vi "Log Status.vi"(7 "Context ID":u32, 8 "error in":errorcluster, 9 "Action":T1, 10 "Socket Counter":u32, 11 "Context Counter":u32) -> (0 "error out":errorcluster)   [LabVIEW 2019, in "RemoteControl.ZMQ.lvlib" / "ZMQ.ContextManager.lvlib"]
uses:
  ZMQ.ContextManager.lvlib
  Typedefs/Action--enum.ctl
  <vilib>/Utility/sysdir.llb/System Directory Type.ctl
  <vilib>/Utility/file.llb/Write Delimited Spreadsheet (string).vi
  <vilib>/Utility/config.llb/Read Key (Boolean).vi
  <vilib>/Utility/config.llb/Write Key (Boolean).vi
  <vilib>/Utility/config.llb/NI_LVConfig.lvlib
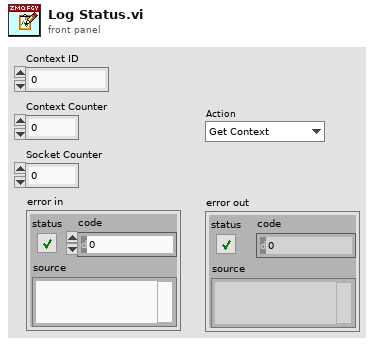
[diagram p1: front panel]
types:
  T1 = typedef "RemoteControl.ZMQ.lvlib/ZMQ.ContextManager.lvlib/Action--enum.ctl" = enum16{"Get Context", "Release Context", "Socket Opened", "Socket Closed", "Force Cleanup"}
  T2 = typedef "System Directory Type.ctl" = i32
  T3 = typedef "NI_LVConfig.lvlib/Config Data RefNum.ctl" = refnum<k1>
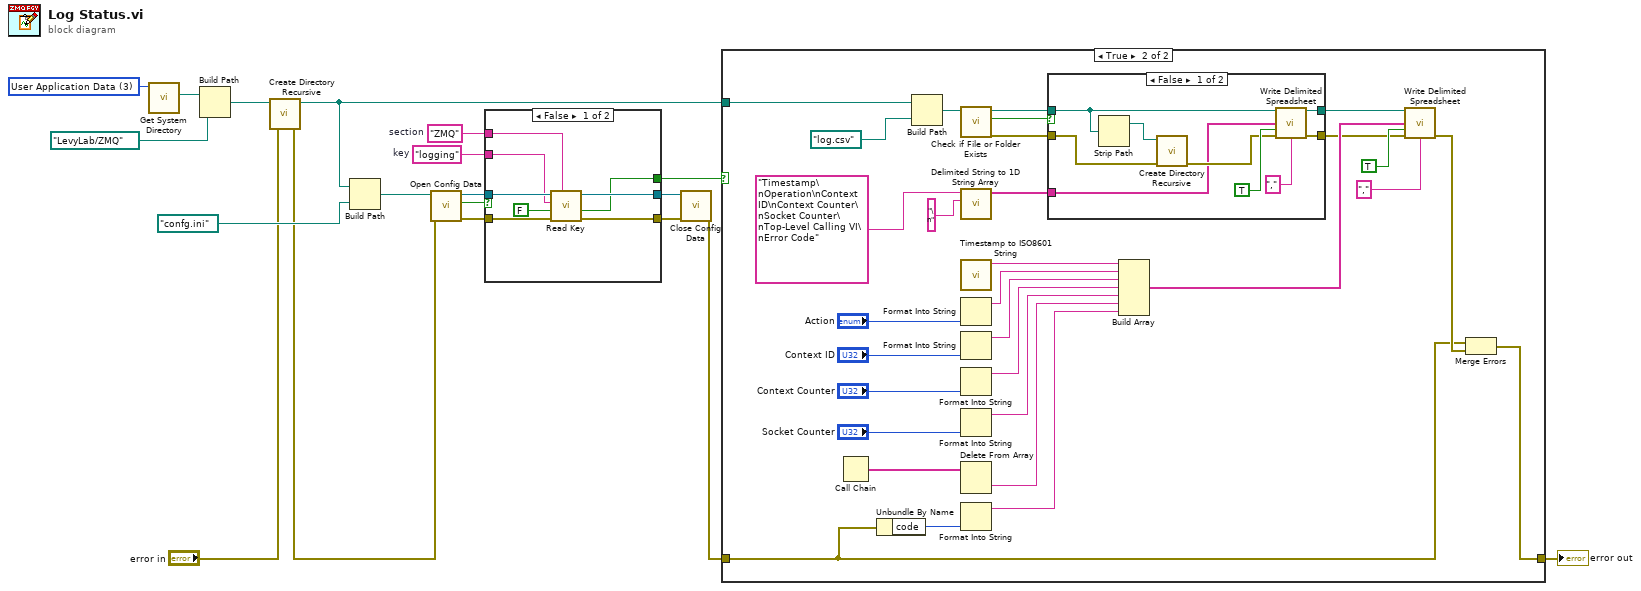
[diagram p0: block diagram]
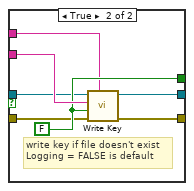
[diagram p2: hidden frame]
diagram:
  w5 = "logging"  # key
  w6 = "ZMQ"  # section
  w19 = T2 3 items=["User Home"=0, "User Desktop"=1, "User Documents"=2, "User Application Data"=3, "User Preferences"=4, "User Temporary"=5, "Public Documents"=6, "Public Application Data"=7, "Public Preferences"=8, "Public Cache"=13, "System Core Libraries"=9, "System Installed Libraries"=10, "Application Files"=11, "Boot Volume Root"=12] ("system directory type")
  n1 = call <vilib>:"Get System Directory.vi"("system directory type"=w19) -> ("system directory"=w18:path)  [unwired: 10 in]
  n2 = Build Path(base path=w18, name or relative path=path "LevyLab/ZMQ") -> (appended path=w4:path)
  n3 = call <vilib>:"Create Directory Recursive.vi"("error in (no error)"="error in", "directory"=w4) -> ("error out"=w1:errorcluster, "directory copy"=w3:path)  [unwired: 3 in, 1 out]
  n4 = Build Path(base path=w3, name or relative path=path "confg.ini") -> (appended path=w15:path)
  n5 = call <vilib>:"Open Config Data.vi"("error in (no error)"=w1, "configuration file path"=w15) -> ("error out"=w13:errorcluster, "file created?"=w7:bool, "refnum"=w14:T3)  [unwired: 7 in]
  n6 = case shown="False" w7 {
    tunnel: w14 -> [w27 w29]
    tunnel: w13 -> [w26 w28]
    tunnel: [w24 w32] -> w11
    tunnel: [w23 w31] -> w10
    tunnel: [w22 w33] -> w8
    tunnel: w6 -> [w21 w30]
    tunnel: w5 -> [w20 w34]
    frame False {
      n7 = call-poly <vilib>:"Read Key.vi"("section"=w21, "error in (no error)"=w26, "default value"=FALSE, "key"=w20, "refnum"=w27) -> ("error out"=w23:errorcluster, "value"=w22:bool, "refnum out"=w24:T3)  [unwired: 3 in, 1 out]
    }
    frame True {
      w33 = FALSE ("value")
      # "write key if file doesn't exist\nLogging = FALSE is default"
      n8 = call-poly <vilib>:"Write Key.vi"("section"=w30, "error in (no error)"=w28, "value"=w33, "key"=w34, "refnum"=w29) -> ("error out"=w31:errorcluster, "refnum out"=w32:T3)  [unwired: 4 in, 1 out]
    }
  }
  n9 = call <vilib>:"Close Config Data.vi"("error in (no error)"=w10, "refnum"=w11) -> ("error out"=w9:errorcluster)  [unwired: 8 in, 1 out]
  n10 = case shown="True" w8 {
    tunnel: w9 -> [w35 w36]
    tunnel: w3 -> [_ w38]
    tunnel: [w35 w37] -> w12
    frame False {
    }
    frame True {
      n11 = Call Chain() -> (call chain=w48:string[])
      n12 = Unbundle By Name(w36) -> ("code"=w54:i32)
      n13 = Build Path(base path=w38, name or relative path=path "log.csv") -> (appended path=w39:path)
      n14 = call <vilib>:"Check if File or Folder Exists.vi"("path"=w39) -> ("error out"=w55:errorcluster, "file or folder exists?"=w62:bool, "dup path"=w63:path)  [unwired: 8 in]
      n15 = call <vilib>:"Delimited String to 1D String Array.vi"("delimiter"="\n", "delimited string"="Timestamp\nOperation\nContext ID\nContext Counter\nSocket Counter\nTop-Level Calling VI\nError Code") -> ("string array"=w64:string[])  [unwired: 9 in]
      n16 = call <vilib>:"Timestamp to ISO8601 String.vi"() -> ("ISO8601 String"=w61:string)  [unwired: 11 in]
      n17 = Format Into String("Action") -> (resulting string=w41:string)  [unwired: 3 in, 1 out]
      n18 = Format Into String("Context ID") -> (resulting string=w42:string)  [unwired: 3 in, 1 out]
      n19 = Format Into String("Context Counter") -> (resulting string=w43:string)  [unwired: 3 in, 1 out]
      n20 = Format Into String("Socket Counter") -> (resulting string=w45:string)  [unwired: 3 in, 1 out]
      n21 = Delete From Array(array=w48) -> (deleted portion=w49:string)  [unwired: 2 in, 1 out]
      n22 = Format Into String(w54) -> (resulting string=w53:string)  [unwired: 3 in, 1 out]
      n23 = case shown="False" w62 {
        tunnel: w64 -> [w66 _]
        tunnel: w63 -> [w71 w75]
        tunnel: [w73 w75] -> w58
        tunnel: [w72 w76] -> w56
        tunnel: w55 -> [w68 w76]
        frame False {
          n24 = Strip Path(path=w71) -> (stripped path=w70:path)  [unwired: 1 out]
          n25 = call <vilib>:"Create Directory Recursive.vi"("error in (no error)"=w68, "directory"=w70) -> ("error out"=w67:errorcluster)  [unwired: 3 in, 2 out]
          n26 = call-poly <vilib>:"Write Delimited Spreadsheet.vi"("file path (dialog if empty)"=w71, "1D data"=w66, "append to file? (new file:F)"=TRUE, "error in (no error)"=w67, "delimiter (\\t)"="," ("delimiter (\\t)")) -> ("new file path (Not A Path if cancelled)"=w73:path, "error out"=w72:errorcluster)  [unwired: 9 in]
        }
        frame True {
        }
      }
      n27 = Build Array(w61, w41, w42, w43, w45, w49, w53) -> (w57:string[])
      n28 = call-poly <vilib>:"Write Delimited Spreadsheet.vi"("file path (dialog if empty)"=w58, "1D data"=w57, "append to file? (new file:F)"=TRUE, "error in (no error)"=w56, "delimiter (\\t)"="," ("delimiter (\\t)")) -> ("error out"=w51:errorcluster)  [unwired: 9 in, 1 out]
      n29 = Merge Errors(w36, w51) -> (w37:errorcluster)
    }
  }
  "error out" <- w12
